vi "alg_transpose (SubVI).vi"(8 "에러 입력(에러 없음)":errorcluster, 11 "matrix":dbl[][](array[numeric])=[[1.0, 1.0]]) -> (0 "에러 출력":errorcluster, 2 "ans":dbl[][](array[numeric]), 3 "참조 번호 출력":refnum<k35>)   [LabVIEW 2018]
uses:
  PythonConfigGlobal.vi
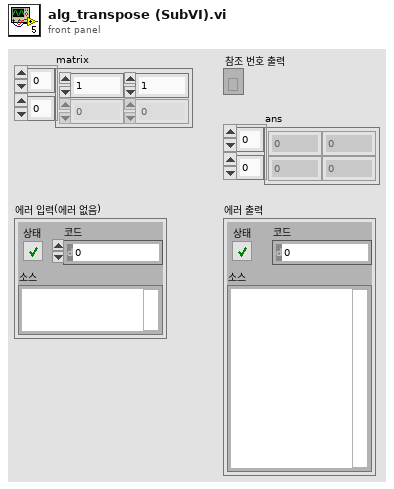
[diagram p1: front panel]
types:
  T1 = cluster{"session out":refnum<k35>, "appended path":path}
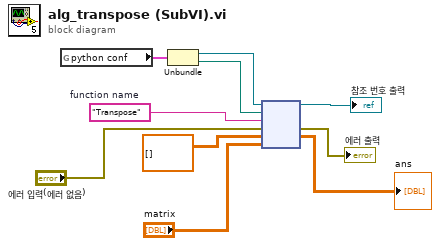
[diagram p0: block diagram]
diagram:
  w9 = "Transpose"  # function name
  n1 = global read "PythonConfigGlobal.vi" "python conf"() -> (w3:T1)
  n2 = Unbundle(w3) -> ("session out"=w5:refnum<k35>, "appended path"=w4:path)
  n3 = node(w5, w4, w9, "에러 입력(에러 없음)", dbl[][] [] ("str1"), "matrix") -> (→"참조 번호 출력":refnum<k35>, →"에러 출력":errorcluster, →"ans":dbl[][])  [unwired: 1 in, 2 out]
